vi "alarm.vi"() -> ()   [LabVIEW 2017]
uses:
  <vilib>/MediaMongrels Ltd/WebSockets/WebSockets/WebSocket Client/WebSocket Client.lvclass
panel:
  out "GetRunState_state":i32
  out "GetAlarmsState_state":dbl[](array[numeric])
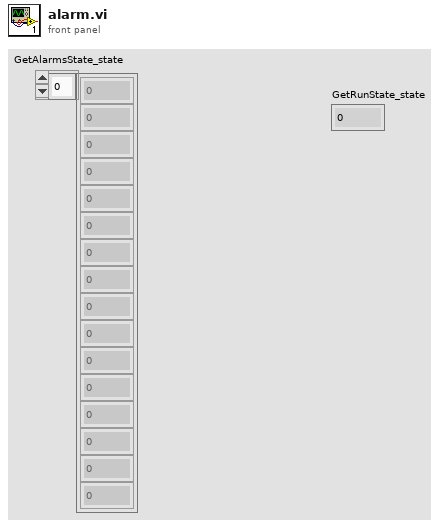
[diagram p1: front panel]
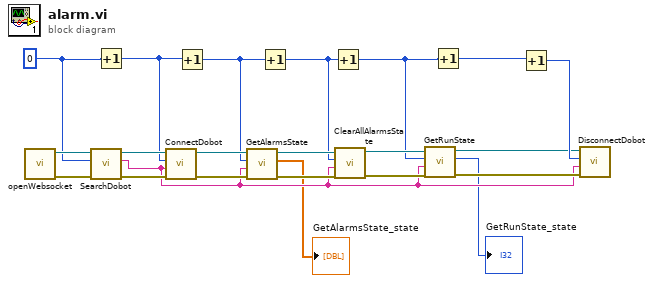
[diagram p0: block diagram]
diagram:
  w18 = 0 ("id")
  n1 = call <vilib>:"openWebsocket.vi"() -> ("error out"=w20:errorcluster, "WebSocket Client out"=w22:refnum<class "WebSocket Client.lvclass">)  [unwired: 10 in]
  n2 = call <vilib>:"SearchDobot.vi"("error in (no error)"=w20, "id"=w18, "WebSocket in"=w22) -> ("error out"=w19:errorcluster, "portName"=w3:string, "WebSocket out"=w21:refnum<class "WebSocket Client.lvclass">)  [unwired: 6 in]
  n3 = Increment(x=w18) -> (x+1=w17:i32)
  n4 = call <vilib>:"ConnectDobot.vi"("error in (no error)"=w19, "portName"=w3, "id"=w17, "WebSocket in"=w21) -> ("error out"=w10:errorcluster, "WebSocket out"=w14:refnum<class "WebSocket Client.lvclass">)  [unwired: 5 in, 1 out]
  n5 = Increment(x=w17) -> (x+1=w6:i32)
  n6 = call <vilib>:"GetAlarmsState.vi"("error in (no error)"=w10, "portName"=w3, "id"=w6, "WebSocket in"=w14) -> ("error out"=w9:errorcluster, "state"=→"GetAlarmsState_state":dbl[], "WebSocket out"=w13:refnum<class "WebSocket Client.lvclass">)  [unwired: 5 in]
  n7 = Increment(x=w6) -> (x+1=w5:i32)
  n8 = Increment(x=w5) -> (x+1=w4:i32)
  n9 = call <vilib>:"ClearAllAlarmsState.vi"("error in (no error)"=w9, "portName"=w3, "id"=w5, "WebSocket in"=w13) -> ("error out"=w8:errorcluster, "WebSocket out"=w12:refnum<class "WebSocket Client.lvclass">)  [unwired: 5 in, 1 out]
  n10 = call <vilib>:"GetRunState.vi"("error in (no error)"=w8, "portName"=w3, "id"=w4, "WebSocket in"=w12) -> ("error out"=w7:errorcluster, "state"=→"GetRunState_state":i32, "WebSocket out"=w11:refnum<class "WebSocket Client.lvclass">)  [unwired: 5 in]
  n11 = Increment(x=w4) -> (x+1=w15:i32)
  n12 = Increment(x=w15) -> (x+1=w16:i32)
  n13 = call <vilib>:"DisconnectDobot.vi"("error in (no error)"=w7, "portName"=w3, "id"=w16, "WebSocket in"=w11) -> ()  [unwired: 5 in, 3 out]
